vi "sensor temperatura DS18B20.vi"(0 "Nombre del puerto serial":refnum<visa-resource-name>="COM1", 1 "baud rate":u32=9600, 2 "bits de datos":u16=8 min=5 max=8 step=1, 3 "paridad":u16(ring) items=["None", "Odd", "Even", "Mark", "Space"], 4 "bits de paro":u16(ring)=10 items=["1.0"=10, "1.5"=15, "2.0"=20], 7 "control de flojo":u16(ring) items=["None"=0, "XON/XOFF"=1, "RTS/CTS"=2, "DTR/DSR"=4]) -> ()   [LabVIEW 2010]
doc: "The Basic Serial Read and Write example performs a Serial Port Read, a Serial Port Write, or a combination of these actions. The user selects the actions (read or write) on the front panel. If both are selected, the VI will write the data first, read data, and then close the VISA session that is opened to the port. This VI will wait until the specified number of bytes is received at the port. Only the number of bytes specified will be read.\n\nINSTRUCTIONS:\n1) Select the serial resource and configuration parameters (baud rate, data bits, parity, stop bits, flow control).\n2) Select the operations to be performed. \n3) Connect the serial port to your device. If no device is available, perform a loopback test by doing one of the following. Short pins 2 and 3 on a RS-232 cable or short pin 4 to pin 8 and pin 5 to pin 9 on a RS-485/422 cable. \n4) Run the VI to see the data read. (The \"read string\" will match the \"string to write\" if a loopback test was performed.)\n\nNote: The parameters set for the serial port must match the parameters of the connected instrument or device. In this example, the bytes to read parameter specifies the number of bytes that the serial port reads. If there were more bytes at the port than the number specified in bytes to read, those bytes would not be read. Also, if you specify to read more bytes than the number of bytes actually read, you might receive a timeout error message.\n\nOn the block diagram, the Configure Serial Port VI sets the configuration parameters. The front panel displays the controls used to configure the basic parameters, such as baud rate, data bits, and parity. Constants configure the other parameters the user probably does not need set. After the VISA Configure Serial Port VI opens the VISA session and configures the port, the VI passes the VISA resource name to other VIs that perform operations on that VISA resource. The VISA Write function sends a command to the serial device and the VISA Read function returns data based on the command. The VISA Close function then closes the reference to the serial device. It is important to close the reference; otherwise communication through with that port through protocols other than VISA might not be possible."
uses:
  <vilib>/Instr/_visa.llb/VISA Configure Serial Port (Instr).vi
panel:
  in  "Tab Control":T1(tab)
  in  "stop 2":bool
  out "°C":dbl(slide) scale=0.0..100.0
  # "Este ejemplo despliega la temperatura en LabView a traves de un puerto COM virtual en windows.\n\nTendras que colocar los archivos de las librerías 1wire.c y DS1820.c en la misma carpeta que tu código de \nprograma CDC_USB_DS18B20.c para poder compilarlo, de lo contrario te marcará error.\n\nDespues de descargar el archivo hex al entrenador, windows lo detectará como nuevo dispositivo usb,\nen ese momento pedira que se instale un driver el cual debera instalarse de forma manual. Este driver\nse encuentra en la carpeta del ejemplo con varias carpetas dependiendo la versión de windows\n\nUna vez instalado el driver, windows instalara un puerto serial COM.\n\nEn el programa de LAbView (con el complemento VISA previamente instalado para que detecte el hardware de la PC)\nseleccionar el puerto serial COM dado de alta en Windows cuando se conectó  el entrenador.\n\nSelecciona la velocidad de transmisión siguiente: 9600bps, 8 bits de datos, 1bit de paro, sin paridad\n\nEjecutar el programa dando un click a la flecha verde y automáticamente se desplegará la información de la \ntemperatura medida por el sensor DS18B20 en el termómetro virtual.\n\nNota: Recuerda colocar una resistencia de PULL-UP de 4.7K en la salida del sensor DS18B20."
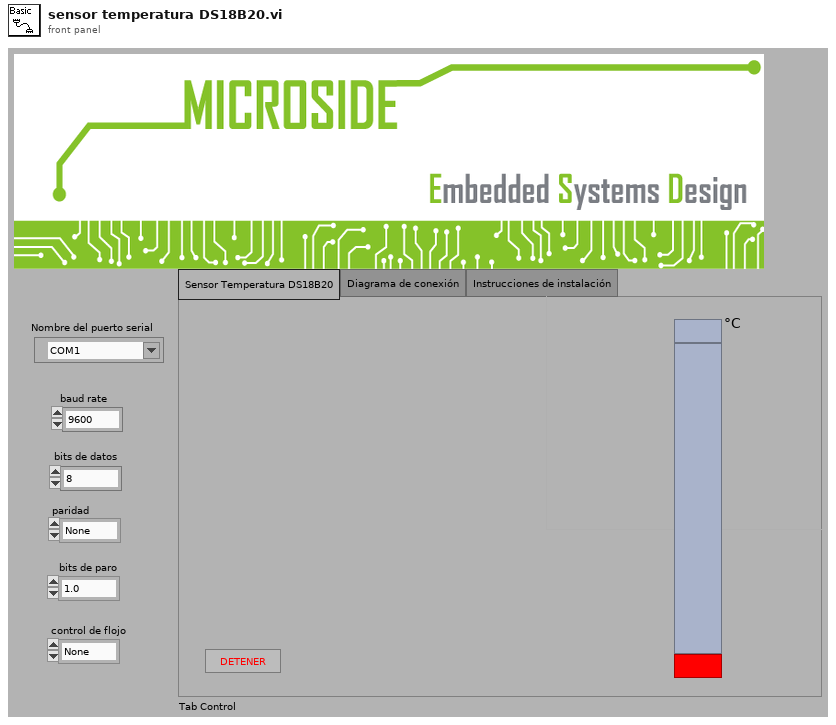
[diagram p1: front panel]
types:
  T1 = enum32{"Sensor Temperatura DS18B20", "Diagrama de conexión", "Instrucciones de instalación"}
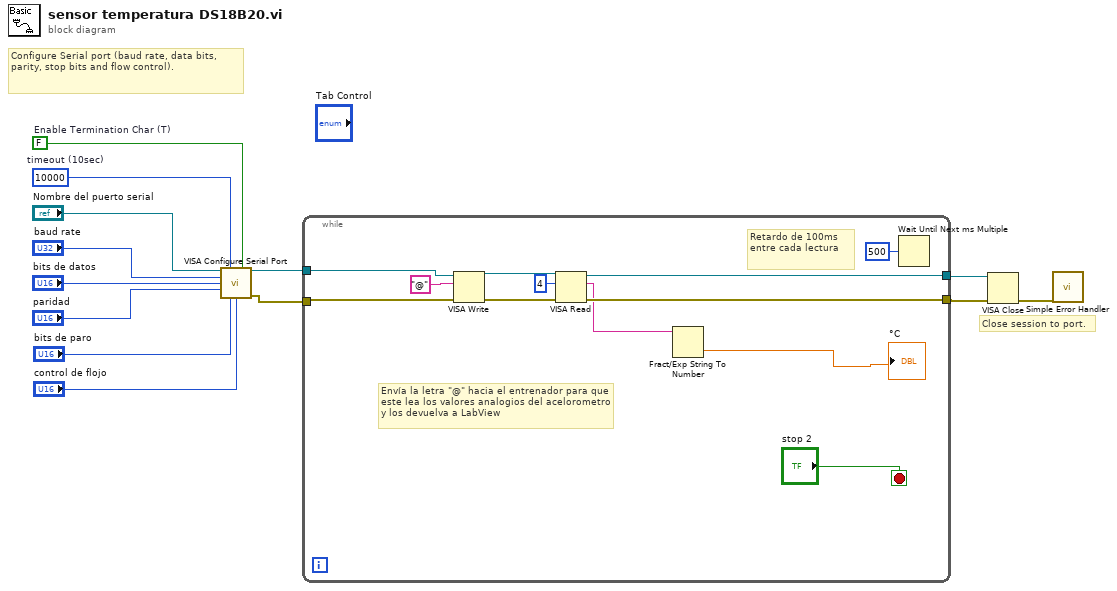
[diagram p0: block diagram]
diagram:
  w8 = FALSE  # Enable Termination Char (T)
  w9 = u32 10000  # timeout (10sec)
  # "Configure Serial port (baud rate, data bits, parity, stop bits and flow control)."
  # "Close session to port."
  n1 = call-poly "VISA Configure Serial Port"("VISA resource name"="Nombre del puerto serial", "timeout (10sec)"=w9, "Enable Termination\nChar (T)"=w8, "baud rate (9600)"="baud rate", "data bits (8)"="bits de datos", "parity (0:none)"="paridad", "stop bits (10: 1 bit)"="bits de paro", "flow control (0:none)"="control de flojo") -> ("VISA resource name out"=w2:refnum<visa-resource-name>, "error out"=w1:errorcluster)  [unwired: 1 in, 5 out]
  n2 = while {
    tunnel: [w22] -> w4
    tunnel: [w21] -> w3
    tunnel: w2 -> [w20]
    tunnel: w1 -> [w17]
    stop <- "stop 2" stop-if-true
    # "Retardo de 100ms entre cada lectura"
    # "Envía la letra \"@\" hacia el entrenador para que este lea los valores analogios del acelorometro y los devuelva a LabView"
    n3 = VISA Write(VISA resource name=w20, write buffer="@" ("string to write 2"), error in (no error)=w17) -> (VISA resource name out=w19:refnum<visa-resource-name>, error out=w18:errorcluster)  [unwired: 1 out]
    n4 = VISA Read(VISA resource name=w19, byte count=u32 4 ("Bytes to Read"), error in (no error)=w18) -> (VISA resource name out=w22:refnum<visa-resource-name>, read buffer=w15:string, error out=w21:errorcluster)  [unwired: 1 out]
    n5 = Fract/Exp String To Number(string=w15) -> (number=→"°C":dbl)  [unwired: 3 in, 1 out]
    n6 = Wait Until Next ms Multiple(millisecond multiple=u32 500) -> ()  [unwired: 1 out]
  }
  n7 = VISA Close(VISA resource name=w4, error in (no error)=w3) -> (error out=w11:errorcluster)
  n8 = call <vilib>:"Simple Error Handler.vi"("error in (no error)"=w11) -> ()  [unwired: 1 in, 8 out]
